vi "Init Actor.vi"(9 "Name Specs":refnum<class "Name Specs.lvclass">, 10 "Project Stuff":refnum<class "Project Stuff.lvclass">) -> (2 "Type":refnum<class "Type.lvclass">)   [LabVIEW 2020, in "_Rescript.lvlib" / "Actor.lvlib"]
uses:
  Actor.lvlib
  Type/Type.lvclass
  _Shared/Name Specs/Name Specs.lvclass
  _Shared/Project Stuff/Project Stuff.lvclass
  Actor/Actor.lvclass
  C:/git/jettl/src/jettl Tools/_Rescript/Type/Type.lvclass
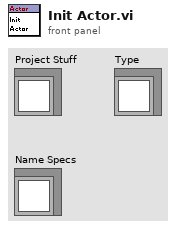
[diagram p1: front panel]
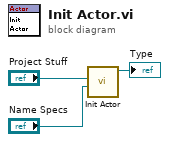
[diagram p0: block diagram]
diagram:
  n1 = call "Init Actor.vi"("Name Specs"="Name Specs", "Project Stuff"="Project Stuff") -> ("Actor out"=→"Type":refnum<class "Actor.lvclass">)  [unwired: 9 in]
